vi "FormatPathArguments.vi"(11 "Arguments":string[](array[string])) -> (3 "Formatted Args":string[](array[string]))   [LabVIEW 2019]
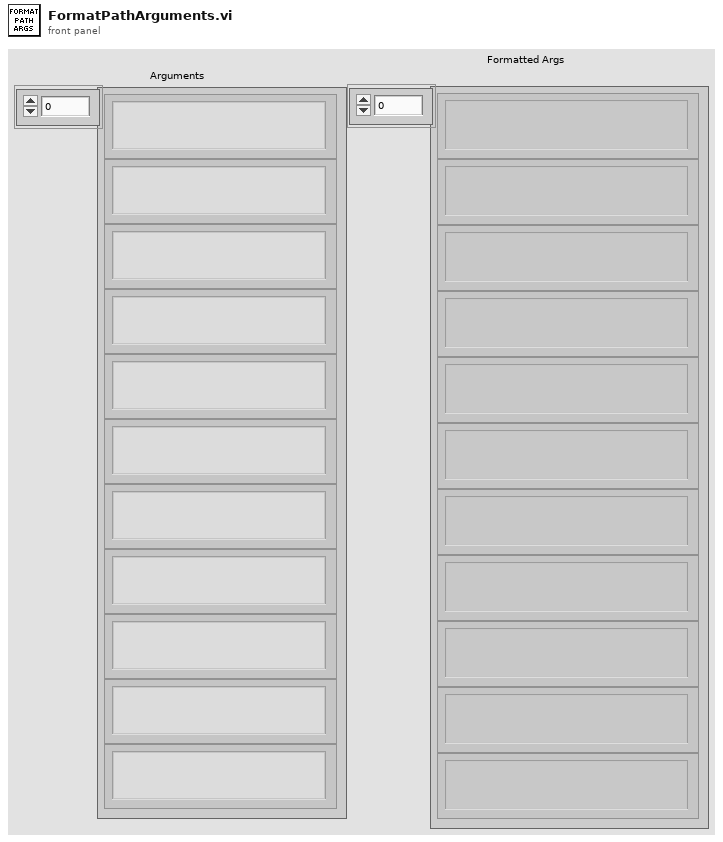
[diagram p1: front panel]
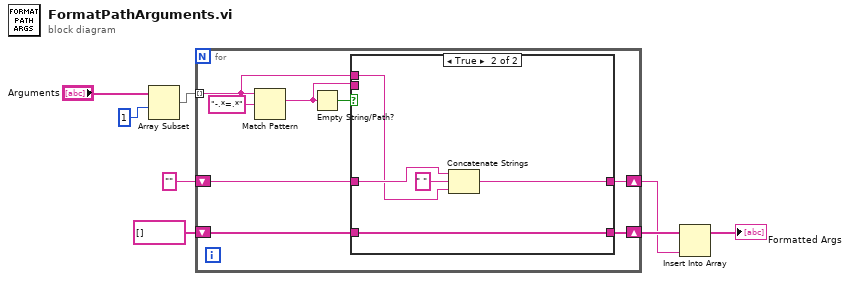
[diagram p0: block diagram]
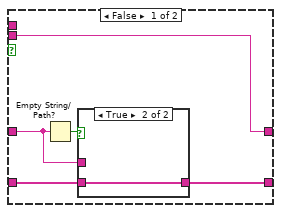
[diagram p2: hidden frame]
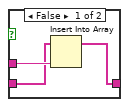
[diagram p3: hidden frame]
diagram:
  n1 = Array Subset(array="Arguments", index=1) -> (w2:string[])  [unwired: 1 in]
  n2 = for {
    tunnel: w2 -> [w9] mode=indexing
    shift-right: [w11] -> w6
    shift-left: string[] [] -> [w12]
    shift-right: [w13] -> w4
    shift-left: "" -> [w14]
    n3 = Match Pattern(string=w9, regular expression="-.*=.*") -> (match substring=w10:string)  [unwired: 1 in, 3 out]
    n4 = Empty String/Path?(string/path=w10) -> (empty?=w15:bool)
    n5 = case shown="True" w15 {
      tunnel: w10 -> [w18 _]
      tunnel: w14 -> [w20 w27]
      tunnel: [w18 w30] -> w13
      tunnel: w12 -> [w17 w29]
      tunnel: [w19 w29] -> w11
      tunnel: w9 -> [_ w26]
      frame False {
        n6 = Empty String/Path?(string/path=w20) -> (empty?=w21:bool)
        n7 = case shown="True" w21 {
          tunnel: w20 -> [w24 _]
          tunnel: w17 -> [w23 w25]
          tunnel: [w22 w25] -> w19
          frame False {
            n8 = Insert Into Array(array=w23, new element=w24) -> (w22:string[])  [unwired: 1 in]
          }
          frame True {
          }
        }
      }
      frame True {
        n9 = Concatenate Strings(w27, " ", w26) -> (w30:string)
      }
    }
  }
  n10 = Insert Into Array(array=w6, new element=w4) -> (→"Formatted Args":string[])  [unwired: 1 in]
